vi "Logic_Config_Device.vi"(4 "error in (no error)":errorcluster, 6 "Device Config":T1={"Enable Digital Channels"=[0, 1, 2, 3], "Digital Sample Rate (Samp/Sec)"=10000000, "Digital Threshold(V)"=3.3000000000000007} {"Digital Threshold(V)" format="%#_13g"; "Digital Sample Rate (Samp/Sec)" format="%.0p"}, 7 "Session Ref In":T2) -> (0 "error out":errorcluster, 1 "Debug Status":string, 3 "Session Ref Out":T2)   [LabVIEW 2023]
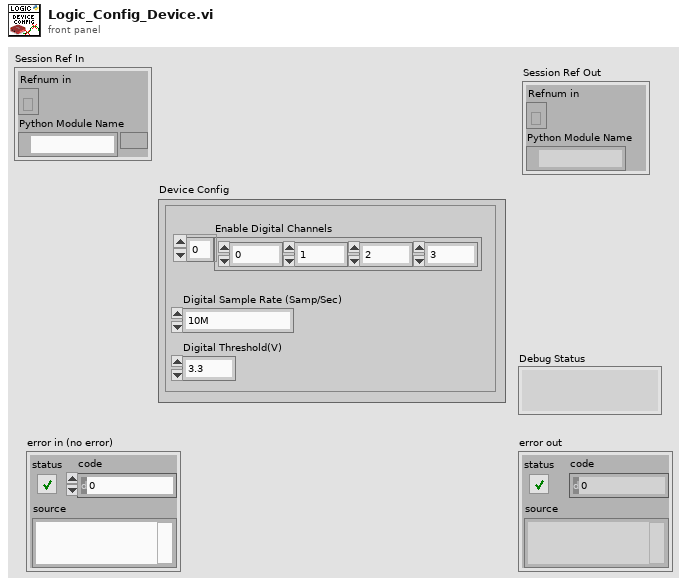
[diagram p1: front panel]
types:
  T1 = cluster{"Enable Digital Channels":i32[], "Digital Sample Rate (Samp/Sec)":i32, "Digital Threshold(V)":dbl}
  T2 = cluster{"Refnum in":refnum<k35>, "Python Module Name":path}
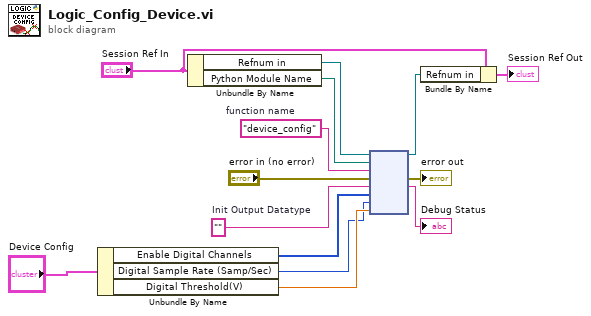
[diagram p0: block diagram]
diagram:
  w12 = "device_config"  # function name
  w11 = ""  # Init Output Datatype
  n1 = Unbundle By Name("Device Config") -> ("Enable Digital Channels"=w3:i32[], "Digital Sample Rate (Samp/Sec)"=w1:i32, "Digital Threshold(V)"=w2:dbl)
  n2 = Unbundle By Name("Session Ref In") -> ("Refnum in"=w9:refnum<k35>, "Python Module Name"=w8:path)
  n3 = node(w9, w8, w12, "error in (no error)", w11, w3, w1, w2) -> (w6:refnum<k35>, →"error out":errorcluster, →"Debug Status":string)  [unwired: 3 in, 2 out]
  n4 = Bundle By Name(cluster="Session Ref In", "Refnum in"=w6) -> (→"Session Ref Out":T2)
